vi "STP_23 - three_multiAO+dynamics+multifreq.vi"() -> ()   [LabVIEW 2020]
uses:
  <vilib>/Utility/error.llb/DialogType.ctl
  <vilib>/measure/NI_MABase.lvlib
  C:/Program Files/National Instruments/LabVIEW 2010/resource/objmgr/daqmx.rc
  <vilib>/Platform/TimedLoop/XDataNode/XDataNode.xnode
  <vilib>/Platform/TimedLoop/XDataNode/nitl_modes.ctl
  <vilib>/Platform/TimedLoop/XDataNode/XDNodeRunTimeDep.lvlib
  <vilib>/Platform/TimedLoop/XDataNode/wakeup.ctl
  <vilib>/Platform/TimedLoop/XDataNode/timing_clust.ctl
  <vilib>/measure/NI_MAPro.lvlib
  <vilib>/Math Plots/2D Math Plots/2D Compass/2D Compass Datatype/2D Compass Datatype.lvclass
  <vilib>/Math Plots/2D Math Plots/2D Compass/2D Compass Datatype/Public/Plot Helper (Vector).vi
  <vilib>/Analysis/NI_AALBase.lvlib
  <vilib>/Analysis/NI_AALPro.lvlib
  <vilib>/measure/matone.llb/Extract Single Tone Information 1 Chan.vi
  <vilib>/DAQmx/write.llb/DAQmx Write (Analog 1D Wfm NChan NSamp).vi
  <vilib>/DAQmx/configure/timing.llb/DAQmx Timing (Sample Clock).vi
  <vilib>/DAQmx/create/timing.llb/DAQmx Create Timing Source (Frequency).vi
  <vilib>/DAQmx/write.llb/DAQmx Write (Analog 2D DBL NChan NSamp).vi
  <vilib>/Instr/_visa.llb/VISA Configure Serial Port (Instr).vi
  <vilib>/DAQmx/create/channels.llb/DAQmx Create Channel (AO-Voltage-Basic).vi
  <vilib>/Math Plots/2D Math Plots/2D Compass/2D Compass XCtrl/2D Compass.xctl
panel:
  in  "Multi-freq. ?":bool
  in  "tones":T1(array[cluster])=[{"frequency"=100.0, "amplitude"=0.1, "phase"=210.0}, {"frequency"=200.0, "amplitude"=0.1, "phase"=39.0}, {"frequency"=250.0, "amplitude"=0.1, "phase"=30.0}, {"frequency"=300.0, "amplitude"=0.1, "phase"=60.0}, {"frequency"=350.0, "amplitude"=0.1, "phase"=184.0}, {"frequency"=400.0, "amplitude"=0.1, "phase"=35.0}] {"phase" format="%.2p"; "amplitude" format="%0.2p"; "frequency" format="%.4p"}
  out "rocof0":dbl[](array[numeric])
  out "rocof1":dbl[](array[numeric])
  out "ROCOF measured":dbl[](array[numeric])
  out "ROCOF reference":dbl[](array[numeric])
  out "Media":dbl
  in  "stop":bool
  out "Frequency reference":dbl[](array[numeric])
  out "Frequency measured":dbl[](array[numeric])
  out "Angle reference":dbl[](array[numeric])
  out "Angle measured":dbl[](array[numeric])
  out "Voltage reference":dbl[](array[numeric])
  out "Voltage measured":dbl[](array[numeric])
  out "freq1":dbl[](array[numeric])
  out "freq0":dbl[](array[numeric])
  out "magnitude1":dbl[](array[numeric])
  out "magnitude0":dbl[](array[numeric])
  in  "last amp":dbl
  out "phases0":dbl[](array[numeric])
  out "phases1":dbl[](array[numeric])
  out "initialized array":dbl[](array[numeric])
  out "Sine phase":dbl
  in  "Tab Control":T2(tab)
  out "Interf.\nAmplitude (%)":dbl
  out "Interf.\nFrequency (Hz)":dbl
  out "Amplitude (%)":dbl
  out "Harmonic order":i32
  out "reset\nphase?":bool
  out "Samples":dbl
  out "Frequency (Hz)":dbl
  out "Phase (deg)":dbl format="%.4f"
  out "Amplitude (V)":dbl format="%.4g"
  in  "Tab Control 3":T3(tab)
  in  "Interference":bool
  in  "Interf. Frequency":dbl caption="Frequency"
  in  "Interf. Amplitude":dbl caption="Amplitude (%)"
  in  "Amplitude (%)":dbl=10.0
  in  "Order":i32=2
  in  "Harmonics":bool
  in  "phase 2":dbl
  in  "duty cycle (%)":dbl=5.0
  in  "Pulse frequency":dbl=25.0
  in  "Noise":bool
  in  "Amplitude":dbl format="%.7f"
  in  "reset signal":bool
  in  "Phase":dbl format="%#.4f"
  in  "Frequency":dbl=50.0 format="%#.4f"
  in  "Offset":dbl=1.5 format="%#.4f"
  in  "Amplitude":dbl=1.25 format="%#.4f"
  in  "Steps":dbl=50.0
  in  "Save without\nvariation":bool
  in  "Amp. (%) 4":dbl=10.0 caption="Amplitude (%)"
  in  "Frequency\ninterval 2":dbl=0.25 caption="Frequency\ninterval"
  in  "Final freq. 2":dbl=51.25 caption="Final freq."
  in  "Initial freq. 2":dbl=48.75 caption="Initial freq."
  in  "Interference\nauto variation":bool
  in  "Amp. (%) 3":dbl=10.0 caption="Amplitude (%)"
  in  "Order\ninterval":i32=1
  in  "Final order":i32=50
  in  "Initial order":i32=2
  in  "Harmonics\nauto variation":bool
  in  "Frequency\ninterval":dbl=0.1 format="%.4f"
  in  "Final freq.":dbl=55.1 format="%.4f"
  in  "Initial freq.":dbl=45.0 format="%.4f"
  in  "Freq. auto\nvariation":bool
  in  "Phase\ninterval":dbl=10.0 format="%.4f"
  in  "Final phase":dbl=180.0 format="%.4f"
  in  "Initial phase":dbl=-180.0 format="%.4f"
  in  "Phase auto\nvariation":bool
  in  "Amplitude\ninterval":dbl=0.1 format="%.4f"
  in  "Initial ampl.":dbl=0.5 format="%.4f"
  in  "Final ampl.":dbl=6.0 format="%.4f"
  in  "Ampl. auto\nvariation":bool
  in  "Modulation tests?":bool
  in  "Final fmod":dbl=2.2
  in  "fmod interval":dbl=0.2
  in  "Initial fmod":dbl
  in  "Modulation\nauto variation":bool
  in  "Select test type":T4(ring)
  in  "Ramp test?":bool
  in  "ka":dbl=0.1
  in  "kx":dbl=0.1
  out "fmod (Hz)":dbl
  in  "fmod":dbl
  in  "Signal generation":bool=TRUE
  in  "File name":path=path "teste.txt"
  in  "Data save":bool
  in  "Boolean":bool
  in  "step time (s)":i32=2
  out "step?":bool
  out "Cycle visualization":dbl[](graph)
  in  "Boolean 3":bool
  out "Phasors visualization":refnum<class "2D Plot Datatype.lvclass">[](xcontrol) caption="2D Compass"
  in  "Directory":path=path "D:/Resultados"
  in  "Sampling rate":dbl=200000.0
  in  "frames per second":dbl=25.0
  in  "Porta":refnum<visa-resource-name>="COM5"
  in  "baud rate (kB)":u32=115200
  in  "data bits (8)":u16=8
  in  "timeout (ms)":u32=5000
  in  "parity (0:none)":enum16{"None", "Odd", "Even", "Mark", "Space"}(ring)
  in  "flow control (0:none)":u16(ring) items=["None", "XON/XOFF", "RTS/CTS", "XON/XOFF & RTS/CTS", "DTR/DSR", "XON/XOFF & DTR/DSR"]
  in  "stop bits (10: 1 bit)":u16(ring)=10 items=["1.0"=10, "1.5"=15, "2.0"=20]
  in  "Serial communication":bool=TRUE
  out "read buffer":string
  out "data":sgl[](array[numeric])
  in  "byte count":u32=16
  in  "Interference 2":bool caption="Interference"
  in  "amplitude":dbl=1.0 caption="Amp. (%)" format="%#.4p"
  in  "Interf. Frequency 2":dbl=10.0 caption="Frequency (Hz)"
  in  "Harmonics 2":bool caption="Harmonics"
  in  "Amp. (%) 2":dbl caption="Amp. (%)"
  in  "Order 2":i32=2 caption="Order"
  out "Frequency":dbl
  in  "Offset 2":dbl=1.5 caption="Offset"
  out "Phase (degrees) 2":dbl caption="Phase (°)" format="%.4f"
  in  "Amplitude 2":dbl=1.25 caption="Amplitude"
  in  "Frequency 2":dbl=50.0 caption="Frequency"
  in  "Phase 2":dbl caption="Phase"
  in  "reset signal 2":bool caption="reset\nsignal"
  in  "Frequency\noff-set":dbl
  in  "Magnitude\noff-set":dbl
  in  "Magnitude\ncoefficient":dbl=1.0
  in  "Angle\noff-set":dbl
  out "mean rocof":dbl caption="ROCOF (Hz/s)" format="%.8g"
  out "max rocof":dbl caption="ROCOF (Hz/s)" format="%.8g"
  out "mean freq":dbl caption="Frequency (Hz)" format="%.8g"
  out "mean tve":dbl caption="TVE (%)" format="%.8g"
  out "mean phase":dbl caption="Phase (º)" format="%.8g"
  out "mean dev":dbl caption="Magnitude (%)" format="%.8g"
  out "max magnitude":dbl caption="Magnitude (%)" format="%.8g"
  out "max tve":dbl caption="TVE (%)" format="%.8g"
  out "max freq":dbl caption="Frequency (Hz)" format="%.8g"
  out "max phase":dbl caption="Phase (º)" format="%.8g"
  in  "Tab Control 2":T5(tab)
  out "Magnitude measures (V)":dbl[][](graph)
  in  "?":bool
  in  "RMS?":bool=TRUE
  out "Phase measures (º)":dbl[][](graph)
  in  "?":bool
  in  "Fase ref":enum16{"R", "S", "T"}(ring)
  out "Frequency measures (Hz)":dbl[][](graph)
  in  "?":bool
  out "ROCOF (Hz/s)":dbl[][](graph)
  in  "?":bool
  in  "?":bool
  out "Phase measures (º) 2":dbl[](graph)
  in  "Index component":i32
  out "Iteration Duration 2":i64
  out "Finished Late? [i-1]":bool
  out "Iteration Duration":i64
  out "Iteration Duration 3":i64
  # "Synchrophasors Test Platform"
  # "A real-time platform for PMU development."
  # "(editar no diagrama de blocos, junto com os dados recebidos)"
  # "Actual generation"
  # "PPS parameters"
  # "Noise"
  # "Sinusoid parameters"
  # "IEEE 754 conversion"
  # "(tamanho do frame)"
  # "Max errors:"
  # "Mean errors:"
  # "Signal generation parameters:"
  # "On-line corrections (received data):"
  # "This is a project developed by Flavio Lori Grando, during Masters in Electrical Engineering Graduate Program (PPGEE) of Federal University of Technology - Paraná, Brazil.\n\nContact: flavio.grando.eng@gmail.com"
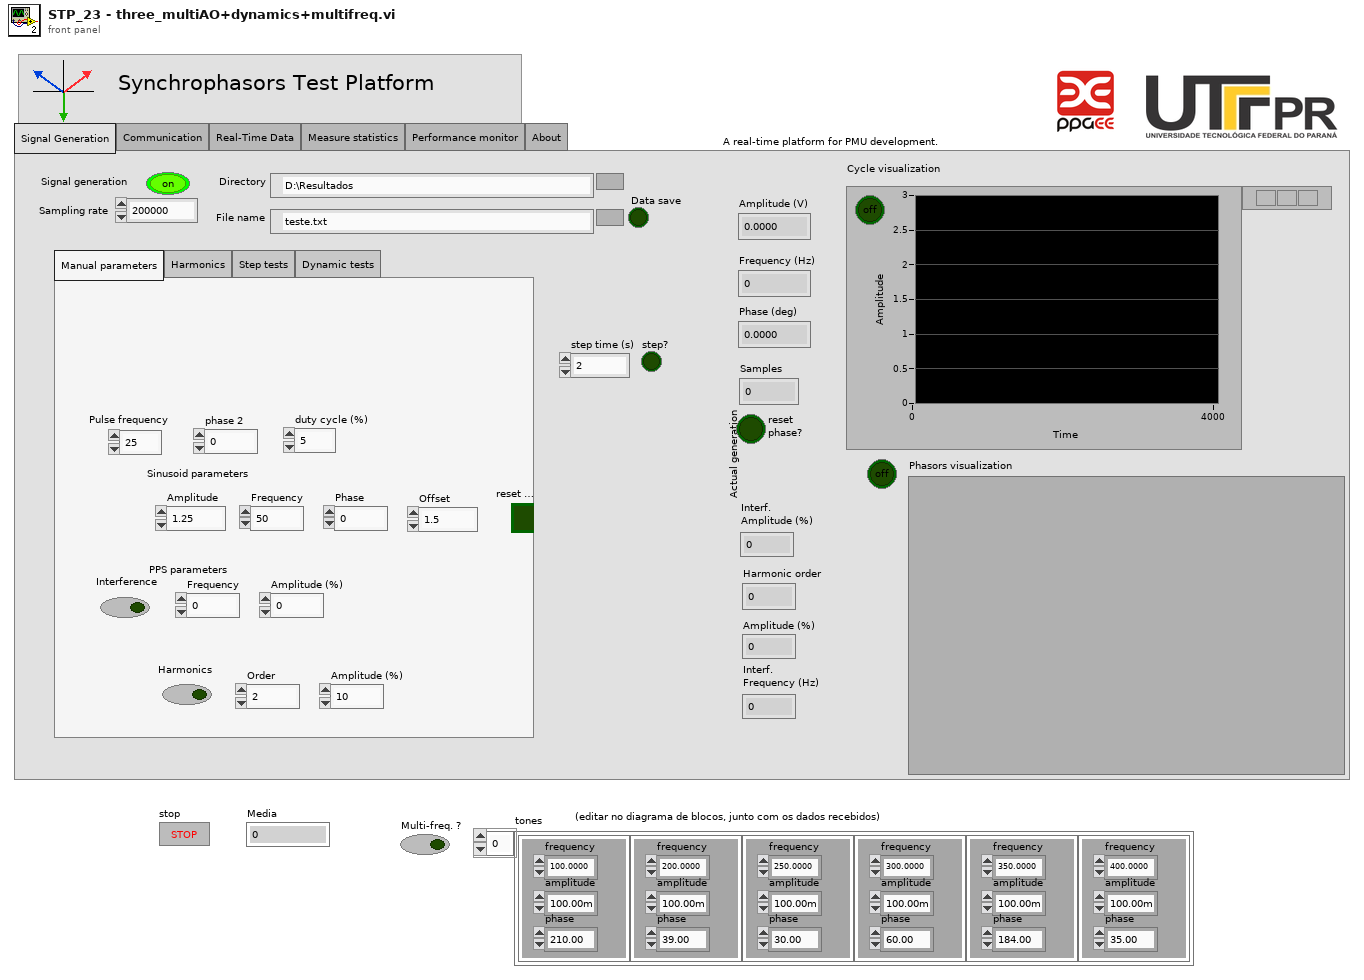
[diagram p1: front panel]
types:
  T1 = cluster{"frequency":dbl, "amplitude":dbl, "phase":dbl}[]
  T2 = enum32{"Signal Generation", "Communication", "Real-Time Data", "Measure statistics", "Performance monitor", "About"}
  T3 = enum32{"Manual parameters", "Harmonics", "Step tests", "Dynamic tests"}
  T4 = enum16{"Amplitude modulation", "Phase modulation", "Frequency ramp"}
  T5 = enum32{"Magnitude", "Phase", "Frequency", "ROCOF", "Phase deviation"}
  T6 = enum16{"Sine Wave", "Triangle Wave", "Square Wave", "Sawtooth Wave"}
  T7 = typedef "XDNodeRunTimeDep.lvlib/nitl_modes.ctl" = enum32{"No Change", "Process missed periods, maintain original phase", "Discard missed periods, maintain original phase", "Process missed periods, ignore original phase", "Discard missed periods, ignore original phase"}
  T8 = typedef "XDNodeRunTimeDep.lvlib/timing_clust.ctl" = cluster{"Expected End [f-1]":u64, "Actual End [f-1]":u64, "Finished Late? [f-1]":bool, "Expected End [i-1]":u64, "Actual End [i-1]":u64, "Finished Late? [i-1]":bool, "Expected Start [i]":u64, "Actual Start [i]":u64, "Expected Start [f]":u64, "Actual Start [f]":u64, "Source Name":string, "Structure Name":string, "Period":i64, "Deadline":i64, "Offset":i64, "Start":i64, "Priority":i32, "Timeout":i32, "Mode":T7, "Wakeup Reason":T9, "Error":errorcluster, "Source Type":string, "Secondary Source Type":string, "Global End Time":u64, "Global Start Time":u64, "Frame Duration":u64, "Iteration Duration":u64, "Assigned CPU":i32, "I/O Scan Engine Mode":u32}
  T9 = typedef "XDNodeRunTimeDep.lvlib/wakeup.ctl" = enum32{"Normal", "Aborted", "Asynchronous wakeup", "Timing source error", "Timed loop error", "Timeout"}
  T10 = typedef "DialogType.ctl" = u16
  T11 = cluster{"Sampling rate":dbl, "Sampling rate":dbl}
  T12 = cluster{"frequency":dbl, "amplitude":dbl, "phase":dbl}
  T13 = enum16{"open", "replace", "create", "open or create", "replace or create", "replace or create with confirmation"}
  T14 = cluster{"max ref":dbl, "min ref":dbl, "mean ref":dbl, "max dev":dbl, "min dev":dbl, "mean dev":dbl, "max meas":dbl, "min meas":dbl, "mean meas":dbl}
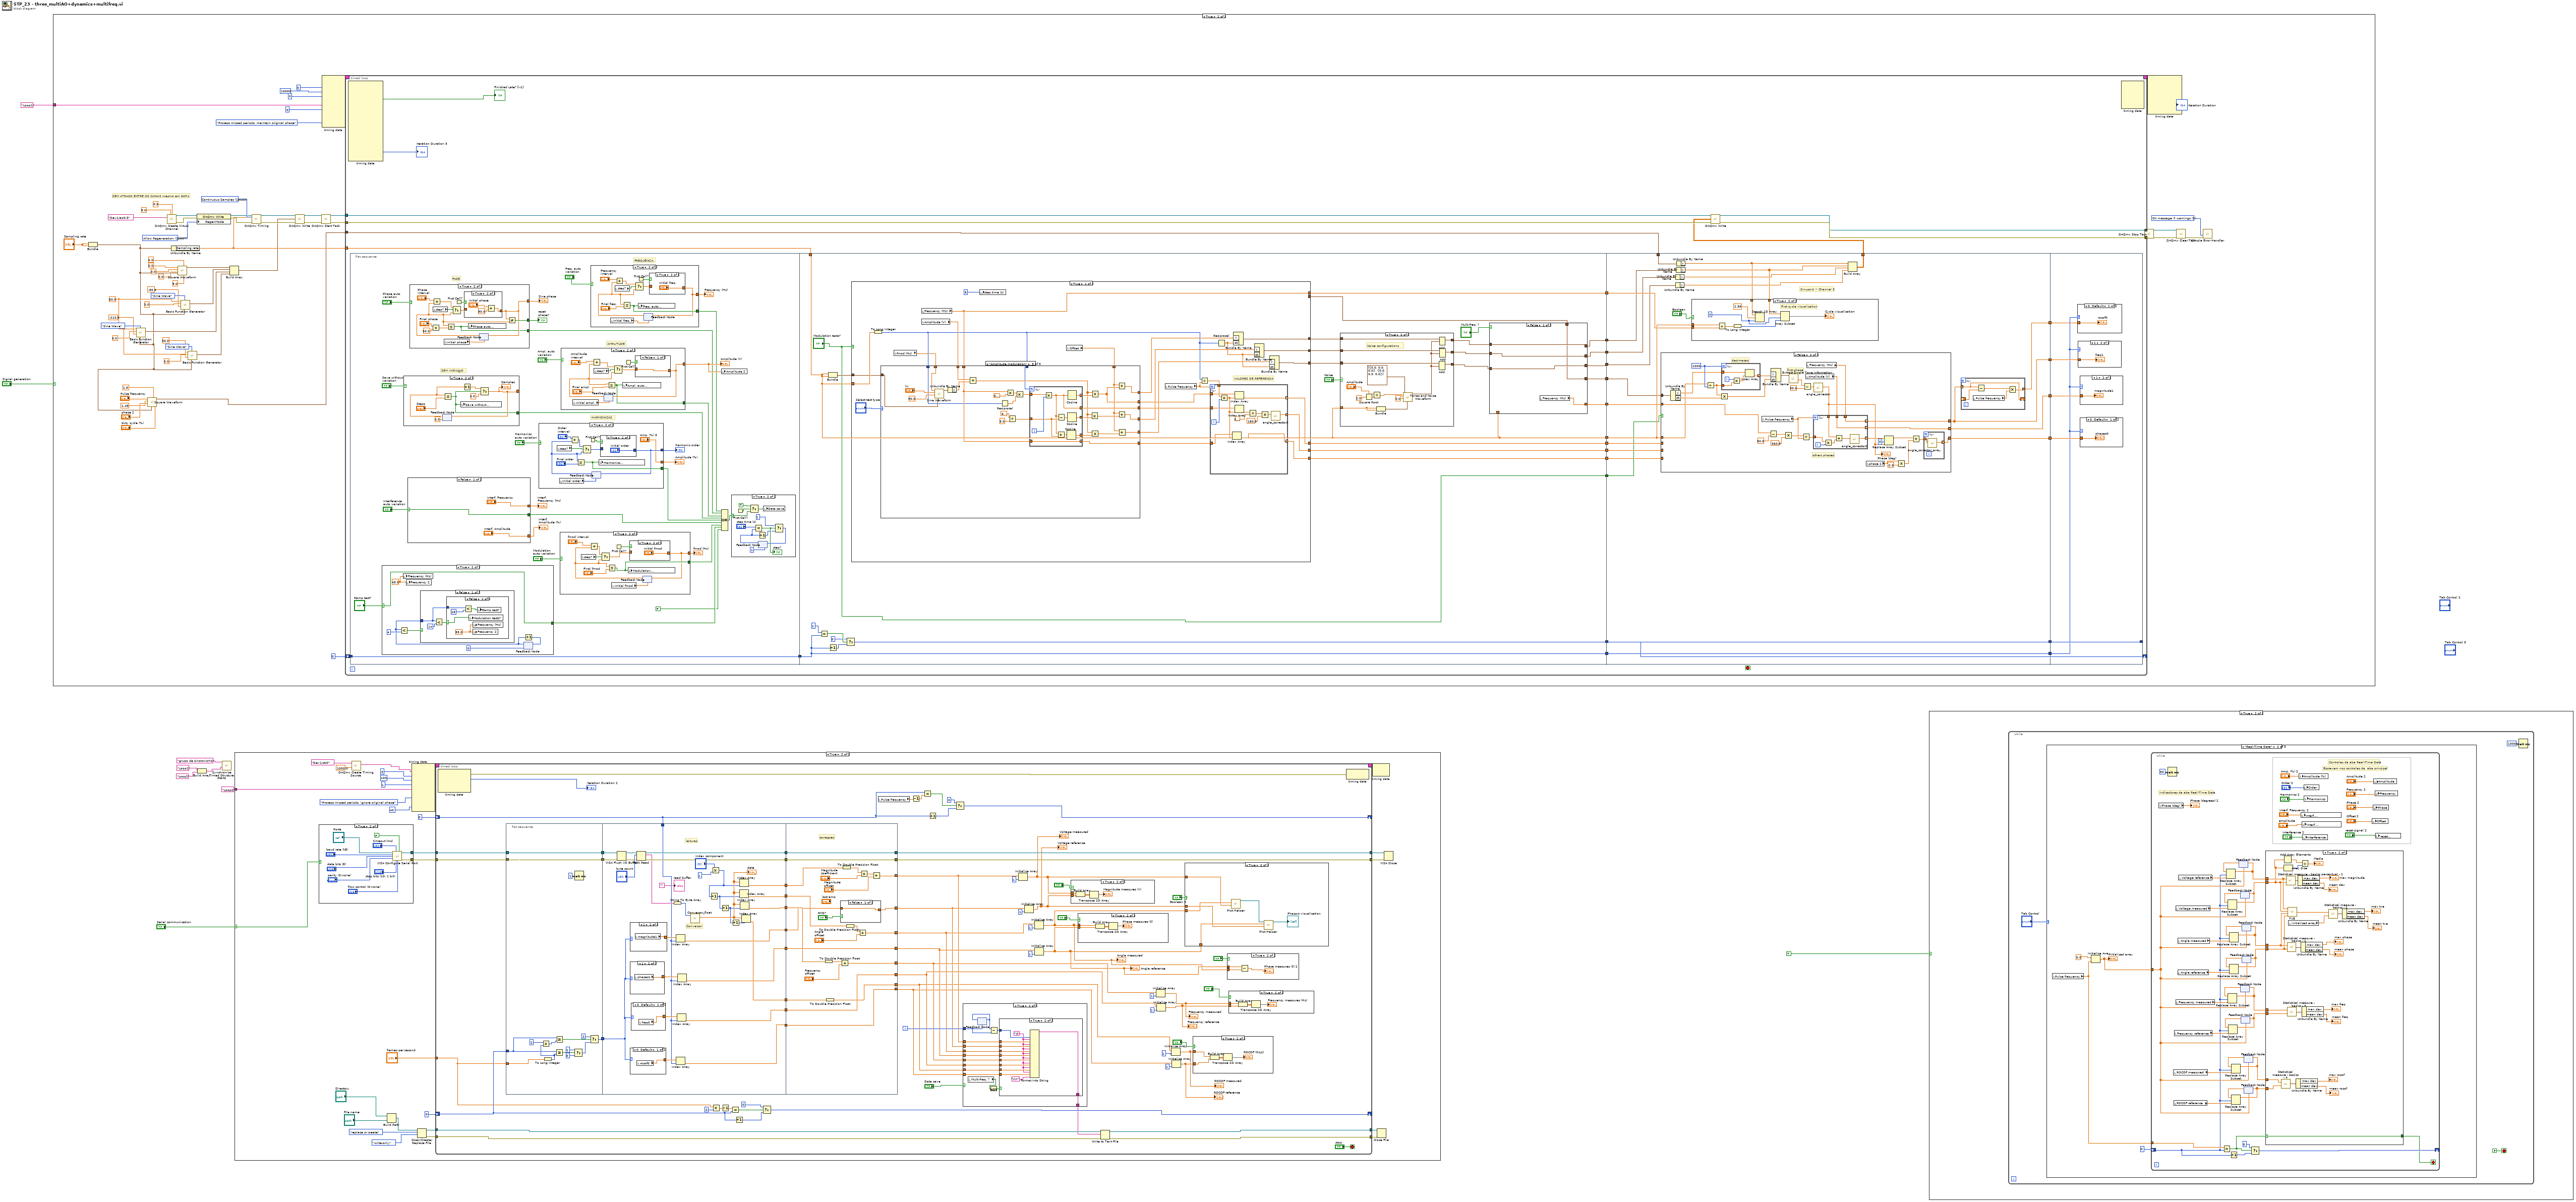
[diagram p0: block diagram]
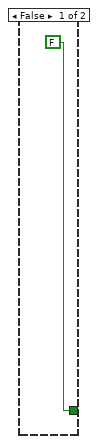
[diagram p4: hidden frame]
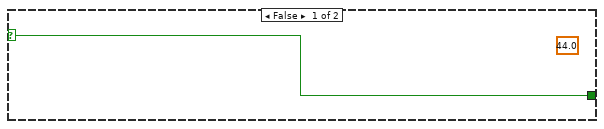
[diagram p7: hidden frame]
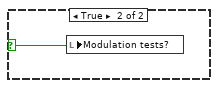
[diagram p8: hidden frame]
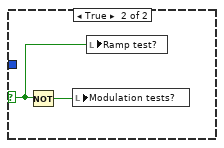
[diagram p9: hidden frame]
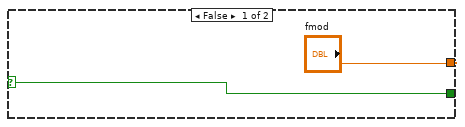
[diagram p10: hidden frame]
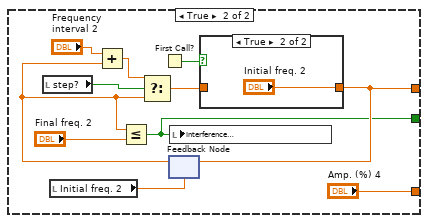
[diagram p12: hidden frame]
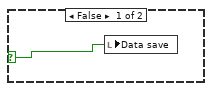
[diagram p14: hidden frame]
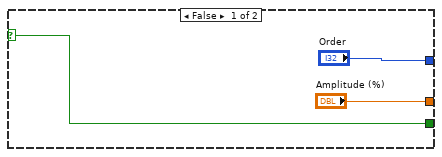
[diagram p15: hidden frame]
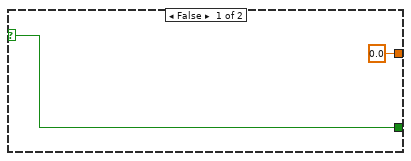
[diagram p17: hidden frame]
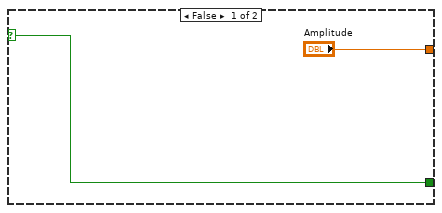
[diagram p18: hidden frame]
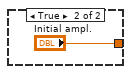
[diagram p19: hidden frame]
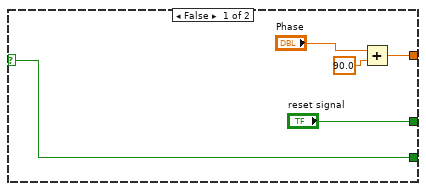
[diagram p20: hidden frame]
diagram:
  n1 = case shown="True" "Signal generation" {
    tunnel: "Loop1" -> [_ w33]
    frame False {
    }
    frame True {
      w20 = 60.0 ("frequency")
      w61 = 10097 items=["Allow Regeneration"=10097, "Do Not Allow Regeneration"=10158] ("RegenMode")
      w64 = 10123 items=["Finite Samples"=10178, "Continuous Samples"=10123] ("sample mode")
      w65 = T10 3 items=["no dialog", "OK message", "continue or stop message", "OK message + warnings", "continue/stop + warnings"] ("type of dialog (OK msg:1)")
      # "SEM ATRASO ENTRE OS CANAIS mesmo em 60Hz"
      n2 = Bundle("Sampling rate"="Sampling rate", "Sampling rate"="Sampling rate") -> (w11:T11)  [unwired: 1 in]
      n3 = call <vilib>:"Basic Function Generator.vi"("sampling info"=w11, "signal type"=T6."Sine Wave" ("signal type 4"), "phase"=-210.0 ("offset 4"), "amplitude"=0.0 ("amplitude 3"), "frequency"=w20) -> ("signal out"=w25:waveform(dbl))  [unwired: 4 in, 2 out]
      n4 = call <vilib>:"Square Waveform.vi"("duty cycle (%)"="duty cycle (%)", "offset"=1.5, "sampling info"=w11, "phase"="phase 2", "amplitude"=1.45, "frequency"="Pulse frequency") -> ("signal out"=w29:waveform(dbl))  [unwired: 4 in, 1 out]
      n5 = call-poly <vilib>:"DAQmx Create Virtual Channel.vi"("maximum value"=3.0 ("Maximum Value"), "minimum value"=0.0 ("Minimum Value"), "physical channels"=tag "Dev1/ao0:3" ("Physical Channel")) -> ("task out"=w40:refnum<k21>, "error out"=w41:errorcluster)  [unwired: 11 in]
      n6 = Unbundle By Name(w11) -> ("Sampling rate"=w10:dbl)
      n7 = call <vilib>:"Square Waveform.vi"("duty cycle (%)"=5.0, "offset"=0.0, "sampling info"=w11, "phase"=0.0, "amplitude"=0.0, "frequency"=0.0) -> ("signal out"=w31:waveform(dbl))  [unwired: 4 in, 1 out]
      n8 = call <vilib>:"Basic Function Generator.vi"("sampling info"=w11, "signal type"=T6."Sine Wave" ("signal type 4"), "phase"=-90.0 ("offset 4"), "amplitude"=0.0 ("amplitude 3"), "frequency"=w20) -> ("signal out"=w32:waveform(dbl))  [unwired: 4 in, 2 out]
      n9 = call <vilib>:"Basic Function Generator.vi"("sampling info"=w11, "signal type"=T6."Sine Wave" ("signal type 4"), "phase"=30.0 ("offset 4"), "amplitude"=0.0 ("amplitude 3"), "frequency"=w20) -> ("signal out"=w21:waveform(dbl))  [unwired: 4 in, 2 out]
      n10 = property class="DAQmx Write"(reference=w40, error in=w41, "RegenMode"=w61) -> (reference out=w14:refnum<k21>, error out=w62:errorcluster)
      n11 = Build Array(w31, w32, w25, w21) -> (w34:waveform(dbl)[])
      n12 = call-poly <vilib>:"DAQmx Timing.vi"("task/channels in"=w14, "sample mode"=w64, "rate"=w10, "error in"=w62) -> ("task out"=w36:refnum<k21>, "error out"=w35:errorcluster)  [unwired: 10 in]
      n13 = call-poly <vilib>:"DAQmx Write.vi"("task/channels in"=w36, "data"=w34, "error in"=w35) -> ("task out"=w45:refnum<k21>, "error out"=w46:errorcluster)  [unwired: 10 in, 1 out]
      n14 = call <vilib>:"DAQmx Start Task.vi"("task/channels in"=w45, "error in"=w46) -> ("task out"=w37:refnum<k21>, "error out"=w38:errorcluster)  [unwired: 12 in]
      n15 = node-c288(i64 0 ("Period"), 10000 ("Priority"), 0 ("Processor"), w33, i64 0 ("Deadline"), nitl_modes."Process missed periods, maintain original phase" ("Mode")) -> (w69:T8)  [unwired: 4 in]
      n16 = timed-loop {
        tunnel: w37 -> [w76]
        tunnel: [w92] -> w54
        tunnel: [w91] -> w53
        timing: w69 -> [_]
        timing-out: [_] -> w68
        shift-right: [w99] -> _
        shift-left: 0 -> [w80]
        tunnel: w38 -> [w93]
        tunnel: w29 -> [w75]
        tunnel: w10 -> [w72]
        stop <- _ stop-if-true
        n17 = node-c288() -> (→"Finished Late? [i-1]":bool, →"Iteration Duration 3":i64)  [unwired: 1 in, 15 out]
        n18 = flat-sequence {
          tunnel: w80 -> [w123]
          tunnel: [w123] -> w89
          tunnel: [w285] -> w90
          tunnel: w89 -> [w284]
          tunnel: [w284] -> w88
          tunnel: [w268] -> w87
          tunnel: [w290] -> w86
          tunnel: [w274] -> w84
          tunnel: [w273] -> w83
          tunnel: [w275] -> w82
          tunnel: [w279] -> w79
          tunnel: [w277] -> w78
          tunnel: [w278] -> w77
          tunnel: ["Modulation tests?"] -> w73
          tunnel: w72 -> [w268]
          tunnel: [w267] -> w71
          tunnel: [w266] -> w70
          tunnel: [w614] -> w98
          tunnel: [w612] -> w97
          tunnel: [w606] -> w96
          tunnel: [w594] -> w95
          tunnel: w90 -> [w614]
          tunnel: w88 -> [w613]
          tunnel: [w613] -> w94
          tunnel: [w609] -> w74
          tunnel: w87 -> [w611]
          tunnel: w86 -> [w610]
          tunnel: [w593] -> w85
          tunnel: w84 -> [w605]
          tunnel: w83 -> [w604]
          tunnel: w82 -> [w599]
          tunnel: w79 -> [w608]
          tunnel: w78 -> [w595]
          tunnel: w77 -> [w607]
          tunnel: w75 -> [w598]
          tunnel: w73 -> [w596]
          tunnel: w71 -> [w592]
          tunnel: w70 -> [w591]
          tunnel: w98 -> [w684]
          tunnel: [w684] -> w99
          tunnel: w97 -> [w683]
          tunnel: w96 -> [w682]
          tunnel: w95 -> [w681]
          tunnel: w94 -> [w680]
          tunnel: w85 -> [w679]
          frame #0 {
            # "HARMONICAS"
            # "SEM VARIA敲O"
            # "FASE"
            # "FREQUÊNCIA"
            # "AMPLITUDE"
            n19 = case shown="True" "Ramp test?" {
              selector: "Ramp test?" -> [w129 w131]
              tunnel: [w129 w131] -> w102
              frame False {
                (unwired) 44.0 ("Initial freq. 3")
              }
              frame True {
                w130 = 45.0 ("Frequency")
                n20 = local write "Frequency (Hz)"(w130) -> ()
                n21 = local write "Frequency 2"(w130) -> ()
                n22 = feedback #1(0) -> (w133:i32)
                n23 = Less?(x=w133, y=4) -> (x < y?=w132:bool)
                n24 = case shown="False" w132 {
                  selector: w132 -> [_ w146]
                  tunnel: w133 -> [w138 _]
                  frame False {
                    n25 = Less?(x=w138, y=14) -> (x < y?=w137:bool)
                    n26 = case shown="False" w137 {
                      selector: w137 -> [w140 w145]
                      tunnel: w138 -> [w143 _]
                      frame False {
                        w141 = 55.0 ("Frequency")
                        n27 = Less?(x=w143, y=18) -> (x < y?=w142:bool)
                        n28 = local write "Modulation tests?"(w140) -> ()
                        n29 = local write "Frequency (Hz)"(w141) -> ()
                        n30 = local write "Frequency 2"(w141) -> ()
                        n31 = local write "Ramp test?"(w142) -> ()
                      }
                      frame True {
                        n32 = local write "Modulation tests?"(w145) -> ()
                      }
                    }
                  }
                  frame True {
                    n33 = Not(x=w146) -> (.not. x?=w147:bool)
                    n34 = local write "Modulation tests?"(w147) -> ()
                    n35 = local write "Ramp test?"(w146) -> ()
                  }
                }
                n36 = Increment(x=w133) -> (x+1=w135:i32)
                n37 = feedback-in #1(w135) -> ()
              }
            }
            n38 = case shown="True" "Save without\nvariation" {
              selector: "Save without\nvariation" -> [w206 _]
              tunnel: [0.0 ("f") w209] -> _
              tunnel: [w206 w208] -> w117
              frame False {
              }
              frame True {
                n39 = feedback #2(0.0 ("f")) -> (w211:dbl)
                n40 = Less Or Equal?(x=w211, y="Steps") -> (x <= y?=w208:bool)
                n41 = local write "Save without\nvariation"(w208) -> ()
                n42 = Increment(x=w211) -> (x+1=w213:dbl)
                n43 = Select(t=w213, s=w208, f=0.0) -> (s? t:f=w209:dbl)
                "Samples" <- w209
                n44 = feedback-in #2(w209) -> ()
              }
            }
            n45 = case shown="False" "Interference\nauto variation" {
              selector: "Interference\nauto variation" -> [w162 _]
              tunnel: ["Interf. Frequency" w171] -> w109
              tunnel: ["Interf. Amplitude" "Amp. (%) 4"] -> w108
              tunnel: [w162 w165] -> w107
              frame False {
              }
              frame True {
                n46 = local read "step?"() -> (w168:bool)
                n47 = local read "Initial freq. 2"() -> (w172:dbl)
                n48 = First Call?() -> (First Call?: T/F=w175:bool)
                n49 = feedback #3(w172) -> (w167:dbl)
                n50 = Add(x="Frequency\ninterval 2", y=w167) -> (x+y=w169:dbl)
                n51 = Less Or Equal?(x=w167, y="Final freq. 2") -> (x <= y?=w165:bool)
                n52 = Select(t=w169, s=w168, f=w167) -> (s? t:f=w174:dbl)
                n53 = local write "Interference\nauto variation"(w165) -> ()
                n54 = case shown="True" w175 {
                  tunnel: [w176 "Initial freq. 2"] -> w171
                  tunnel: w174 -> [w176 _]
                  frame False {
                  }
                  frame True {
                  }
                }
                n55 = feedback-in #3(w171) -> ()
              }
            }
            "Interf.\nFrequency (Hz)" <- w109
            "Interf.\nAmplitude (%)" <- w108
            n56 = case shown="True" "Phase auto\nvariation" {
              selector: "Phase auto\nvariation" -> [w229 _]
              tunnel: ["reset signal" w244] -> w128
              tunnel: [w231 w243] -> w118
              tunnel: [w229 w238] -> w115
              frame False {
                n57 = Add(x="Phase", y=90.0) -> (x+y=w231:dbl)
              }
              frame True {
                n58 = Add(x="Final phase", y=90.0) -> (x+y=w240:dbl)
                n59 = local read "step?"() -> (w234:bool)
                n60 = local read "Initial phase"() -> (w242:dbl)
                n61 = First Call?() -> (First Call?: T/F=w245:bool)
                n62 = feedback #4(w242) -> (w236:dbl)
                n63 = Add(x="Phase\ninterval", y=w236) -> (x+y=w235:dbl)
                n64 = Less Or Equal?(x=w236, y=w240) -> (x <= y?=w238:bool)
                n65 = Select(t=w235, s=w234, f=w236) -> (s? t:f=w237:dbl)
                n66 = case shown="True" w245 {
                  tunnel: [w247 w248] -> w243
                  tunnel: w237 -> [w247 _]
                  frame False {
                  }
                  frame True {
                    n67 = Add(x="Initial phase", y=90.0) -> (x+y=w248:dbl)
                  }
                }
                n68 = local write "Phase auto\nvariation"(w238) -> ()
                n69 = feedback-in #4(w243) -> ()
                n70 = Not Equal?(x=w243, y=w236) -> (x != y?=w244:bool)
              }
            }
            "Sine phase" <- w118
            "reset\nphase?" <- w128
            n71 = case shown="True" "Harmonics\nauto variation" {
              selector: "Harmonics\nauto variation" -> [w191 _]
              tunnel: ["Order" w197] -> w113
              tunnel: [w191 w198] -> w111
              tunnel: ["Amplitude (%)" "Amp. (%) 3"] -> w112
              frame False {
              }
              frame True {
                n72 = local read "step?"() -> (w200:bool)
                n73 = local read "Initial order"() -> (w202:i32)
                n74 = First Call?() -> (First Call?: T/F=w199:bool)
                n75 = feedback #5(w202) -> (w195:i32)
                n76 = Add(x="Order\ninterval", y=w195) -> (x+y=w194:i32)
                n77 = Less Or Equal?(x=w195, y="Final order") -> (x <= y?=w198:bool)
                n78 = Select(t=w194, s=w200, f=w195) -> (s? t:f=w203:i32)
                n79 = local write "Harmonics\nauto variation"(w198) -> ()
                n80 = case shown="True" w199 {
                  tunnel: [w204 "Initial order"] -> w197
                  tunnel: w203 -> [w204 _]
                  frame False {
                  }
                  frame True {
                  }
                }
                n81 = feedback-in #5(w197) -> ()
              }
            }
            "Harmonic order" <- w113
            "Amplitude (%)" <- w112
            n82 = case shown="True" "Modulation\nauto variation" {
              selector: "Modulation\nauto variation" -> [w149 _]
              tunnel: [w149 w152] -> w105
              tunnel: ["fmod" w151] -> w104
              frame False {
              }
              frame True {
                n83 = local read "step?"() -> (w158:bool)
                n84 = local read "Initial fmod"() -> (w150:dbl)
                n85 = First Call?() -> (First Call?: T/F=w159:bool)
                n86 = feedback #6(w150) -> (w155:dbl)
                n87 = Add(x="fmod interval", y=w155) -> (x+y=w157:dbl)
                n88 = Select(t=w157, s=w158, f=w155) -> (s? t:f=w153:dbl)
                n89 = Less Or Equal?(x=w155, y="Final fmod") -> (x <= y?=w152:bool)
                n90 = local write "Modulation\nauto variation"(w152) -> ()
                n91 = case shown="True" w159 {
                  tunnel: [w160 "Initial fmod"] -> w151
                  tunnel: w153 -> [w160 _]
                  frame False {
                  }
                  frame True {
                  }
                }
                n92 = feedback-in #6(w151) -> ()
              }
            }
            "fmod (Hz)" <- w104
            n93 = case shown="True" "Ampl. auto\nvariation" {
              selector: "Ampl. auto\nvariation" -> [w215 _]
              tunnel: ["Amplitude" w224] -> w122
              tunnel: [w215 w219] -> w116
              frame False {
              }
              frame True {
                n94 = local read "Initial ampl."() -> (w223:dbl)
                n95 = local read "step?"() -> (w220:bool)
                n96 = feedback #7(w223) -> (w218:dbl)
                n97 = Add(x="Amplitude\ninterval", y=w218) -> (x+y=w222:dbl)
                n98 = Less Or Equal?(x=w218, y="Final ampl.") -> (x <= y?=w219:bool)
                n99 = Select(t=w222, s=w220, f=w218) -> (s? t:f=w221:dbl)
                n100 = local write "Ampl. auto\nvariation"(w219) -> ()
                n101 = First Call?() -> (First Call?: T/F=w225:bool)
                n102 = case shown="False" w225 {
                  tunnel: [w227 "Initial ampl."] -> w224
                  tunnel: w221 -> [w227 _]
                  frame False {
                  }
                  frame True {
                  }
                }
                n103 = feedback-in #7(w224) -> ()
              }
            }
            "Amplitude (V)" <- w122
            n104 = case shown="True" "Freq. auto\nvariation" {
              selector: "Freq. auto\nvariation" -> [w252 _]
              tunnel: ["Frequency" w259] -> w120
              tunnel: [w252 w257] -> w114
              frame False {
              }
              frame True {
                n105 = local read "Initial freq."() -> (w258:dbl)
                n106 = local read "step?"() -> (w253:bool)
                n107 = First Call?() -> (First Call?: T/F=w261:bool)
                n108 = feedback #8(w258) -> (w254:dbl)
                n109 = Add(x="Frequency\ninterval", y=w254) -> (x+y=w255:dbl)
                n110 = Less Or Equal?(x=w254, y="Final freq.") -> (x <= y?=w257:bool)
                n111 = Select(t=w255, s=w253, f=w254) -> (s? t:f=w256:dbl)
                n112 = local write "Freq. auto\nvariation"(w257) -> ()
                n113 = case shown="True" w261 {
                  tunnel: [w263 "Initial freq."] -> w259
                  tunnel: w256 -> [w263 _]
                  frame False {
                  }
                  frame True {
                  }
                }
                n114 = feedback-in #8(w259) -> ()
              }
            }
            "Frequency (Hz)" <- w120
            n115 = local write "Amplitude 2"(w122) -> ()
            n116 = Compound Arithmetic op=OR(w114, w115, w116, w117, w111, w107, w105, w102, FALSE ("Boolean 2")) -> (w119:bool)
            n117 = case shown="True" w119 {
              selector: w119 -> [w178 w187]
              frame False {
                n118 = local write "Data save"(w178) -> ()
              }
              frame True {
                n119 = First Call?() -> (First Call?: T/F=w189:bool)
                n120 = Select(t=TRUE, s=w189, f=w187) -> (s? t:f=w186:bool)
                n121 = feedback #9(1 ("f")) -> (w179:i32)
                n122 = Equal?(x="step time (s)", y=w179) -> (x = y?=w182:bool)
                "step?" <- w182
                n123 = Increment(x=w179) -> (x+1=w180:i32)
                n124 = local write "Data save"(w186) -> ()
                n125 = Select(t=1 ("f"), s=w182, f=w180) -> (s? t:f=w185:i32)
                n126 = feedback-in #9(w185) -> ()
              }
            }
          }
          frame #1 {
            n127 = Equal?(x=1, y=w284) -> (x = y?=w289:bool)
            n128 = Bundle("Sampling rate"=w268, "Sampling rate"=w268) -> (w291:T11)  [unwired: 1 in]
            n129 = Increment(x=w284) -> (x+1=w287:i32)
            n130 = Select(t=0, s=w289, f=w287) -> (s? t:f=w285:i32)
            n131 = case shown="True" "Modulation tests?" {
              tunnel: w291 -> [w342 w521]
              tunnel: [w346 w537] -> w290
              tunnel: [w351 w519] -> w283
              tunnel: [w350 w520] -> w282
              tunnel: [w356 w518] -> w280
              tunnel: [_ w523] -> w265
              tunnel: w268 -> [w354 _]
              tunnel: [w345 _] -> w279
              tunnel: [w344 _] -> w278
              tunnel: [w335 _] -> w277
              frame True {
                # "VALORES DE REFERENCIA"
                n132 = To Long Integer(number=w354) -> (32bit integer=w348:i32)
                n133 = local read "fmod (Hz)"() -> (w343:dbl)
                n134 = local read "Frequency (Hz)"() -> (w346:dbl)
                n135 = local read "Amplitude (V)"() -> (w355:dbl)
                n136 = local write "step time (s)"(5) -> ()
                n137 = local read "Offset"() -> (w334:dbl)
                n138 = case shown="\"Amplitude modulation\"" "Select test type" {
                  tunnel: w355 -> [w368 w413 w493]
                  tunnel: w346 -> [w365 w411 w481]
                  tunnel: w348 -> [_ w416 w474]
                  tunnel: [w382 w402 w488] -> w336
                  tunnel: [w362 w408 w465] -> w339
                  tunnel: [w360 w403 w467] -> w341
                  tunnel: [w359 w405 w469] -> w340
                  tunnel: w348 -> [w364 _ w471]
                  tunnel: [w376 w415 w480] -> w337
                  tunnel: w343 -> [w374 _ w475]
                  tunnel: w342 -> [w375 _ w473]
                  tunnel: [w367 w419 w464] -> w338
                  tunnel: w334 -> [w358 w407 w468]
                  frame "Phase modulation" {
                    # "referencia"
                    n139 = call <vilib>:"Sine Waveform.vi"("sampling info"=w375, "phase"=-90.0, "amplitude"="ka", "frequency"=w374) -> ("signal out"=w378:waveform(dbl))  [unwired: 6 in, 1 out]
                    n140 = call <vilib>:"Sine Waveform.vi"("sampling info"=w375, "phase"=-180.0, "amplitude"="ka", "frequency"=w374) -> ("signal out"=w372:waveform(dbl))  [unwired: 6 in, 1 out]
                    n141 = Unbundle By Name(w378) -> ("Y"=w369:dbl[])
                    n142 = Unbundle By Name(w372) -> ("Y"=w371:dbl[])
                    n143 = Reciprocal(x=w364) -> (1/x=w366:dbl)
                    n144 = Multiply(x=w365, y=6.283185307179586) -> (x*y=w380:dbl)
                    n145 = Divide(x=6.283185307179586, y=3.0) -> (x/y=w385:dbl)
                    n146 = Multiply(x=w380, y=w366) -> (x*y=w381:dbl)
                    n147 = for {
                      N: w364 -> [_]
                      tunnel: w381 -> [w393]
                      tunnel: [w401] -> w388 mode=indexing
                      tunnel: [w390] -> w382 mode=indexing
                      tunnel: w385 -> [w398]
                      tunnel: [w397] -> w384 mode=indexing
                      tunnel: [w396] -> w383 mode=indexing
                      tunnel: w369 -> [w390] mode=indexing
                      tunnel: [w391] -> w367 mode=indexing
                      tunnel: w368 -> [w391]
                      i -> [w392]
                      n148 = Multiply(x=w393, y=w392) -> (x*y=w395:dbl)
                      n149 = Add(x=w395, y=w390) -> (x+y=w394:dbl)
                      n150 = Add(x=w394, y=w398) -> (x+y=w399:dbl)
                      n151 = Subtract(x=w394, y=w398) -> (x-y=w400:dbl)
                      n152 = Cosine(x=w399) -> (cos(x)=w397:dbl)
                      n153 = Cosine(x=w400) -> (cos(x)=w396:dbl)
                      n154 = Cosine(x=w394) -> (cos(x)=w401:dbl)
                    }
                    n155 = Multiply(x=w371, y=w374) -> (x*y=w377:dbl[])
                    n156 = Multiply(x=w368, y=w383) -> (x*y=w361:dbl[])
                    n157 = Multiply(x=w368, y=w384) -> (x*y=w357:dbl[])
                    n158 = Multiply(x=w368, y=w388) -> (x*y=w363:dbl[])
                    n159 = Subtract(x=w365, y=w377) -> (x-y=w376:dbl[])
                    n160 = Add(x=w358, y=w363) -> (x+y=w362:dbl[])
                    n161 = Add(x=w358, y=w357) -> (x+y=w359:dbl[])
                    n162 = Add(x=w358, y=w361) -> (x+y=w360:dbl[])
                  }
                  frame "Frequency ramp" {
                    w422 = u16 0 items=["2nd Order Central", "4th Order Central", "Forward", "Backward"] ("method")
                    w417 = 1 items=["none", "linear"] ("interpolation")
                    w428 = cluster{"Fs":dbl, "#s":dbl} {"Fs"=25000.0, "#s"=25000.0} ("sampling info")
                    n163 = case shown="True" TRUE {
                      tunnel: w416 -> [w438 w456]
                      tunnel: [w435 w453] -> w415
                      tunnel: w411 -> [w439 w451]
                      frame False {
                        n164 = First Call?() -> (First Call?: T/F=w441:bool)
                        n165 = feedback #10(w439) -> (w442:dbl)
                        n166 = Decrement(x=w442) -> (x-1=w440:dbl)
                        n167 = Select(t=w439, s=w441, f=w440) -> (s? t:f=w443:dbl)
                        n168 = feedback-in #10(w443) -> ()
                        n169 = Reciprocal(x=w438) -> (1/x=w436:dbl)
                        n170 = for {
                          N: w438 -> [_]
                          tunnel: w436 -> [w447]
                          tunnel: [w446] -> w444 mode=indexing
                          i -> [w445]
                          n171 = Multiply(x=w447, y=w445) -> (x*y=w446:dbl)
                        }
                        n172 = Subtract(x=w443, y=w444) -> (x-y=w437:dbl[])
                        n173 = Subtract(x=w437, y=w436) -> (x-y=w435:dbl[])
                      }
                      frame True {
                        w448 = 1.0 ("x")
                        n174 = First Call?() -> (First Call?: T/F=w458:bool)
                        n175 = feedback #11(w451) -> (w450:dbl)
                        n176 = Add(x=w448, y=w450) -> (x+y=w449:dbl)
                        n177 = Select(t=w451, s=w458, f=w449) -> (s? t:f=w457:dbl)
                        n178 = feedback-in #11(w457) -> ()
                        n179 = Reciprocal(x=w456) -> (1/x=w452:dbl)
                        n180 = for {
                          N: w456 -> [_]
                          tunnel: w452 -> [w463]
                          tunnel: [w460] -> w455 mode=indexing
                          tunnel: w448 -> [w459]
                          i -> [w462]
                          n181 = Multiply(x=w463, y=w462) -> (x*y=w461:dbl)
                          n182 = Multiply(x=w459, y=w461) -> (x*y=w460:dbl)
                        }
                        n183 = Add(x=w457, y=w455) -> (x+y=w454:dbl[])
                        n184 = Add(x=w452, y=w454) -> (x+y=w453:dbl[])
                      }
                    }
                    n185 = call <vilib>:"Formula Waveform.vi"("sampling info"=w428, "formula"="a*cos(w*t+pi(1)*t*t)", "amplitude"=w413, "frequency"=w411) -> ("signal out"=w433:waveform(dbl))  [unwired: 6 in, 1 out]
                    n186 = call <vilib>:"Formula Waveform.vi"("sampling info"=w428, "formula"="a*cos(w*t+pi(1)*t*t-pi(1)*2/3)", "amplitude"=w413, "frequency"=w411) -> ("signal out"=w430:waveform(dbl))  [unwired: 6 in, 1 out]
                    n187 = call <vilib>:"Formula Waveform.vi"("sampling info"=w428, "formula"="a*cos(w*t+pi(1)*t*t+2*pi(1)/3)", "amplitude"=w413, "frequency"=w411) -> ("signal out"=w429:waveform(dbl))  [unwired: 6 in, 1 out]
                    n188 = Unbundle By Name(w430) -> ("Y"=w425:dbl[])
                    n189 = Unbundle By Name(w429) -> ("Y"=w424:dbl[])
                    n190 = Unbundle By Name(w433) -> ("Y"=w426:dbl[])
                    n191 = Divide(x=1.0, y=w416) -> (x/y=w423:dbl)
                    n192 = call <vilib>:"Arbitrary Wave.vi"("interpolation"=w417, "Wave Table"=w426, "frequency"=w423, "samples"=w416) -> ("arbitrary wave"=w409:dbl[])  [unwired: 3 in, 2 out]
                    n193 = call <vilib>:"Arbitrary Wave.vi"("interpolation"=w417, "Wave Table"=w424, "frequency"=w423, "samples"=w416) -> ("arbitrary wave"=w406:dbl[])  [unwired: 3 in, 2 out]
                    n194 = call <vilib>:"Arbitrary Wave.vi"("interpolation"=w417, "Wave Table"=w425, "frequency"=w423, "samples"=w416) -> ("arbitrary wave"=w404:dbl[])  [unwired: 3 in, 2 out]
                    n195 = Divide(x=w409, y=w413) -> (x/y=w412:dbl[])
                    n196 = Inverse Cosine(1:w412) -> (0:w414:dbl[])
                    n197 = Initialize Array(w413, w416) -> (w419:dbl[])
                    n198 = call <vilib>:"Derivative x(t).vi"("method"=w422, "dt"=1e-05, "X"=w414) -> ("dX/dt"=w420:dbl[])  [unwired: 7 in, 1 out]
                    n199 = Sign(1:w420) -> (0:w418:dbl[])
                    n200 = Multiply(x=w414, y=w418) -> (x*y=w402:dbl[])
                    n201 = Add(x=w407, y=w409) -> (x+y=w408:dbl[])
                    n202 = Add(x=w407, y=w404) -> (x+y=w403:dbl[])
                    n203 = Add(x=w407, y=w406) -> (x+y=w405:dbl[])
                  }
                  frame "Amplitude modulation" {
                    n204 = call <vilib>:"Sine Waveform.vi"("sampling info"=w473, "phase"=90.0 ("phase in"), "amplitude"="kx", "frequency"=w475) -> ("signal out"=w477:waveform(dbl))  [unwired: 6 in, 1 out]
                    n205 = Unbundle By Name(w477) -> ("Y"=w476:dbl[])
                    n206 = Add(x=w493, y=w476) -> (x+y=w482:dbl[])
                    n207 = Reciprocal(x=w471) -> (1/x=w472:dbl)
                    n208 = Multiply(x=w481, y=6.283185307179586) -> (x*y=w491:dbl)
                    n209 = Divide(x=6.283185307179586, y=3.0) -> (x/y=w485:dbl)
                    n210 = Multiply(x=w491, y=w472) -> (x*y=w490:dbl)
                    n211 = for {
                      N: w474 -> [_]
                      tunnel: w490 -> [w501]
                      tunnel: [w502] -> w489 mode=indexing
                      tunnel: [w498] -> w488 mode=indexing
                      tunnel: w485 -> [w497]
                      tunnel: [w496] -> w484 mode=indexing
                      tunnel: [w495] -> w483 mode=indexing
                      tunnel: [w494] -> w480 mode=indexing
                      tunnel: w481 -> [w494]
                      i -> [w503]
                      n212 = Multiply(x=w501, y=w503) -> (x*y=w498:dbl)
                      n213 = Add(x=w498, y=w497) -> (x+y=w499:dbl)
                      n214 = Subtract(x=w498, y=w497) -> (x-y=w500:dbl)
                      n215 = Cosine(x=w499) -> (cos(x)=w496:dbl)
                      n216 = Cosine(x=w500) -> (cos(x)=w495:dbl)
                      n217 = Cosine(x=w498) -> (cos(x)=w502:dbl)
                    }
                    n218 = Multiply(x=w482, y=w483) -> (x*y=w466:dbl[])
                    n219 = Multiply(x=w482, y=w484) -> (x*y=w470:dbl[])
                    n220 = Multiply(x=w482, y=w489) -> (x*y=w464:dbl[])
                    n221 = Add(x=w468, y=w464) -> (x+y=w465:dbl[])
                    n222 = Add(x=w468, y=w466) -> (x+y=w467:dbl[])
                    n223 = Add(x=w468, y=w470) -> (x+y=w469:dbl[])
                  }
                }
                n224 = local read "Pulse frequency"() -> (w353:dbl)
                n225 = Divide(x=w348, y=w353) -> (x/y=w352:dbl)
                n226 = for {
                  N: w353 -> [_]
                  tunnel: w336 -> [w517]
                  tunnel: w352 -> [w515]
                  tunnel: [w508] -> w345 mode=indexing
                  tunnel: w338 -> [w509]
                  tunnel: [w507] -> w344 mode=indexing
                  tunnel: w337 -> [w506]
                  tunnel: [w504] -> w335 mode=indexing
                  i -> [w516]
                  n227 = Multiply(x=w515, y=w516) -> (x*y=w505:dbl)
                  n228 = Index Array(array=w506, index=w505) -> (element=w504:dbl)
                  n229 = Index Array(array=w517, index=w505) -> (element=w512:dbl)
                  n230 = Index Array(array=w509, index=w505) -> (element=w508:dbl)
                  n231 = Divide(x=w512, y=3.141592653589793) -> (x/y=w511:dbl)
                  n232 = Multiply(x=w511, y=180.0) -> (x*y=w510:dbl)
                  n233 = call "angle_corrector2.vi"("angle"=w510) -> ("angle corrected"=w507:dbl)  [unwired: 10 in]
                }
                n234 = Reciprocal(x=w348) -> (1/x=w349:dbl)
                n235 = Bundle By Name("Y"=w339, "dt"=w349) -> (w356:waveform(dbl))  [unwired: 1 in]
                n236 = Bundle By Name("Y"=w341, "dt"=w349) -> (w351:waveform(dbl))  [unwired: 1 in]
                n237 = Bundle By Name("Y"=w340, "dt"=w349) -> (w350:waveform(dbl))  [unwired: 1 in]
              }
              frame False {
                # "Sinusoid configurations"
                n238 = local read "reset\nphase?"() -> (w536:bool)
                n239 = local read "Frequency (Hz)"() -> (w537:dbl)
                n240 = local read "Amplitude (V)"() -> (w538:dbl)
                n241 = local read "Sine phase"() -> (w542:dbl)
                n242 = local write "Offset 2"("Offset") -> ()
                n243 = Subtract(x=w542, y=120.0) -> (x-y=w544:dbl)
                n244 = call <vilib>:"Sine Waveform.vi"("offset"="Offset", "sampling info"=w521, "reset signal"=w536, "phase"=w542, "amplitude"=w538, "frequency"=w537) -> ("signal out"=w526:waveform(dbl))  [unwired: 4 in, 1 out]
                n245 = Subtract(x=w542, y=240.0) -> (x-y=w541:dbl)
                n246 = call <vilib>:"Sine Waveform.vi"("offset"="Offset", "sampling info"=w521, "reset signal"=w536, "phase"=w544, "amplitude"=w538, "frequency"=w537) -> ("signal out"=w525:waveform(dbl))  [unwired: 4 in, 1 out]
                n247 = call <vilib>:"Sine Waveform.vi"("offset"="Offset", "sampling info"=w521, "reset signal"=w536, "phase"=w541, "amplitude"=w538, "frequency"=w537) -> ("signal out"=w524:waveform(dbl))  [unwired: 4 in, 1 out]
                n248 = case shown="\"R\"" "Fase ref" {
                  tunnel: w526 -> [_ _ w549]
                  tunnel: w525 -> [w547 _ _]
                  tunnel: w524 -> [_ w548 _]
                  tunnel: [w547 w548 w549] -> w523
                  frame "S" {
                  }
                  frame "T" {
                  }
                  frame "R" {
                  }
                }
                n249 = local read "Harmonics\nauto variation"() -> (w532:bool)
                n250 = local read "Amplitude (V)"() -> (w531:dbl)
                n251 = Or(x=w532, y="Harmonics") -> (x .or. y?=w534:bool)
                n252 = case shown="True" w534 {
                  tunnel: w524 -> [w572 w585]
                  tunnel: [w572 w584] -> w546
                  tunnel: w521 -> [_ w583]
                  tunnel: w525 -> [w571 w581]
                  tunnel: w526 -> [w570 w580]
                  tunnel: [w571 w578] -> w540
                  tunnel: [w570 w577] -> w539
                  tunnel: [w569 w574] -> w535
                  tunnel: w531 -> [w569 w574]
                  frame False {
                  }
                  frame True {
                    n253 = local read "Amplitude (%)"() -> (w576:dbl)
                    n254 = local read "Harmonic order"() -> (w582:i32)
                    n255 = local read "Frequency (Hz)"() -> (w575:dbl)
                    n256 = Divide(x=w576, y=100.0) -> (x/y=w587:dbl)
                    n257 = Multiply(x=w575, y=w582) -> (x*y=w590:dbl)
                    "Frequency" <- w590
                    n258 = Multiply(x=w574, y=w587) -> (x*y=w586:dbl)
                    n259 = call <vilib>:"Sine Waveform.vi"("sampling info"=w583, "phase"=180.0, "amplitude"=w586, "frequency"=w590) -> ("error out"=w573:errorcluster, "signal out"=w579:waveform(dbl))  [unwired: 6 in]
                    n260 = Add(1:w579, 2:w580, 4:w573) -> (0:w577:waveform(dbl))  [unwired: 1 out]
                    n261 = Add(1:w579, 2:w581, 4:w573) -> (0:w578:waveform(dbl))  [unwired: 1 out]
                    n262 = Add(1:w579, 2:w585, 4:w573) -> (0:w584:waveform(dbl))  [unwired: 1 out]
                  }
                }
                n263 = local read "Interference\nauto variation"() -> (w528:bool)
                n264 = Or(x="Interference", y=w528) -> (x .or. y?=w530:bool)
                n265 = case shown="True" w530 {
                  tunnel: w535 -> [_ w565]
                  tunnel: w521 -> [_ w564]
                  tunnel: w546 -> [w552 w563]
                  tunnel: [w552 w562] -> w520
                  tunnel: w540 -> [w551 w561]
                  tunnel: w539 -> [w550 w559]
                  tunnel: [w551 w560] -> w519
                  tunnel: [w550 w557] -> w518
                  frame False {
                  }
                  frame True {
                    n266 = local read "Interf.\nFrequency (Hz)"() -> (w555:dbl)
                    n267 = local read "Interf.\nAmplitude (%)"() -> (w556:dbl)
                    n268 = Divide(x=w556, y=100.0) -> (x/y=w567:dbl)
                    n269 = Multiply(x=w565, y=w567) -> (x*y=w566:dbl)
                    n270 = call <vilib>:"Sine Waveform.vi"("sampling info"=w564, "phase"=0.0, "amplitude"=w566, "frequency"=w555) -> ("error out"=w553:errorcluster, "signal out"=w558:waveform(dbl))  [unwired: 6 in]
                    n271 = Add(1:w558, 2:w561, 4:w553) -> (0:w560:waveform(dbl))  [unwired: 1 out]
                    n272 = Add(1:w558, 2:w559, 4:w553) -> (0:w557:waveform(dbl))  [unwired: 1 out]
                    n273 = Add(1:w558, 2:w563, 4:w553) -> (0:w562:waveform(dbl))  [unwired: 1 out]
                  }
                }
              }
            }
            n274 = case shown="True" "Noise" {
              tunnel: w283 -> [w316 w332]
              tunnel: w280 -> [w317 w331]
              tunnel: [w317 w330] -> w270
              tunnel: [w316 w329] -> w271
              tunnel: [w315 w328] -> w272
              tunnel: w282 -> [w315 w327]
              tunnel: w268 -> [_ w323]
              frame False {
              }
              frame True {
                # "Noise configurations"
                n275 = Square Root(x=2.0 ("offset")) -> (sqrt(x)=w320:dbl)
                n276 = Divide(x="Amplitude", y=w320) -> (x/y=w318:dbl)
                n277 = Bundle("Sampling rate"=w323, "Sampling rate"=w323) -> (w326:T11)  [unwired: 1 in]
                n278 = call <vilib>:"Tones and Noise Waveform.vi"("sampling info"=w326, "offset"=0.0, "noise (rms)"=w318, "tones"=T1 [{"frequency"=0.0, "amplitude"=0.0, "phase"=0.0}, {"frequency"=0.0, "amplitude"=0.0, "phase"=0.0}]) -> ("signal out"=w322:waveform(dbl))  [unwired: 6 in, 1 out]
                n279 = Add(1:w322, 2:w327) -> (0:w328:waveform(dbl))  [unwired: 1 in, 1 out]
                n280 = Add(1:w322, 2:w331) -> (0:w330:waveform(dbl))  [unwired: 1 in, 1 out]
                n281 = Add(1:w322, 2:w332) -> (0:w329:waveform(dbl))  [unwired: 1 in, 1 out]
              }
            }
            n282 = case shown="False" "Multi-freq. ?" {
              tunnel: w270 -> [w296 w310]
              tunnel: w272 -> [w295 w309]
              tunnel: [w295 w307] -> w273
              tunnel: [w294 w306] -> w274
              tunnel: [w296 w305] -> w275
              tunnel: w271 -> [w294 w304]
              tunnel: w268 -> [_ w302]
              tunnel: [w292 w301] -> w267
              tunnel: [w293 w298] -> w266
              tunnel: w265 -> [w292 _]
              frame False {
                n283 = local read "Frequency (Hz)"() -> (w293:dbl)
              }
              frame True {
                # "para gerar referencias"
                n284 = Square Root(x=2.0 ("offset")) -> (sqrt(x)=w314:dbl)
                n285 = Bundle("Sampling rate"=w302, "Sampling rate"=w302) -> (w303:T11)  [unwired: 1 in]
                n286 = Divide(x=0.0, y=w314) -> (x/y=w312:dbl)
                n287 = call <vilib>:"Tones and Noise Waveform.vi"("sampling info"=w303, "noise (rms)"=w312, "tones"="tones") -> ("error out"=w308:errorcluster, "signal out"=w301:waveform(dbl))  [unwired: 7 in]
                n288 = Index Array(array="tones", index=0) -> (element=w299:T12)
                n289 = Add(1:w301, 2:w310, 4:w308) -> (0:w305:waveform(dbl))  [unwired: 1 out]
                n290 = Add(1:w301, 2:w304, 4:w308) -> (0:w306:waveform(dbl))  [unwired: 1 out]
                n291 = Add(1:w301, 2:w309, 4:w308) -> (0:w307:waveform(dbl))  [unwired: 1 out]
                n292 = Unbundle By Name(w299) -> ("frequency"=w298:dbl)
              }
            }
          }
          frame #2 {
            # "Sinusoid > Channel 3"
            n293 = case shown="False" w596 {
              tunnel: [w631 w646] -> w606
              tunnel: [w630 w633] -> w612
              tunnel: w611 -> [_ w645]
              tunnel: [w629 w644] -> w594
              tunnel: w592 -> [_ w639]
              tunnel: w608 -> [w631 _]
              tunnel: w595 -> [w629 _]
              tunnel: w607 -> [w630 _]
              tunnel: w591 -> [_ w632]
              frame True {
              }
              frame False {
                w660 = 1000
                # "others phases"
                # "first phase"
                # "decimacao"
                n294 = Unbundle By Name(w639) -> ("Y"=w640:dbl[], "dt"=w641:dbl)
                n295 = Divide(x=w645, y=w660) -> (x/y=w659:dbl)
                n296 = Multiply(x=w659, y=w641) -> (x*y=w662:dbl)
                n297 = for {
                  N: w660 -> [_]
                  tunnel: w640 -> [w678]
                  tunnel: [w675] -> w663 mode=indexing
                  tunnel: w659 -> [w674]
                  i -> [w676]
                  n298 = Multiply(x=w676, y=w674) -> (x*y=w677:dbl)
                  n299 = Index Array(array=w678, index=w677) -> (element=w675:dbl)
                }
                n300 = local read "Pulse frequency"() -> (w650:dbl)
                n301 = Subtract(x=w632, y=50.0) -> (x-y=w653:dbl)
                n302 = Bundle By Name("Y"=w663, "dt"=w662) -> (w661:waveform(dbl))  [unwired: 1 in]
                n303 = Multiply(x=w653, y=360.0) -> (x*y=w652:dbl)
                n304 = call-poly <vilib>:"Extract Single Tone Information.vi"("time signal in"=w661) -> ("detected phase (deg)"=w657:dbl)  [unwired: 5 in, 5 out]
                n305 = Divide(x=w652, y=w650) -> (x/y=w649:dbl)
                n306 = Subtract(x=w657, y=90.0) -> (x-y=w656:dbl)
                n307 = local read "Amplitude (V)"() -> (w643:dbl)
                n308 = local read "Frequency (Hz)"() -> (w642:dbl)
                n309 = call "angle_corrector.vi"("angle"=w656) -> ("angle corrected"=w647:dbl)  [unwired: 10 in]
                "Phase (deg)" <- w647
                n310 = for {
                  N: w650 -> [_]
                  tunnel: [w667] -> w651 mode=indexing
                  tunnel: w649 -> [w671]
                  tunnel: w647 -> [w672]
                  tunnel: w643 -> [w669]
                  tunnel: [w669] -> w646 mode=indexing
                  tunnel: w642 -> [w668]
                  tunnel: [w668] -> w644 mode=indexing
                  i -> [w673]
                  n311 = Multiply(x=w671, y=w673) -> (x*y=w670:dbl)
                  n312 = Add(x=w672, y=w670) -> (x+y=w666:dbl)
                  n313 = call "angle_corrector2.vi"("angle"=w666) -> ("angle corrected"=w667:dbl)  [unwired: 10 in]
                }
                n314 = local read "phase 2"() -> (w636:dbl)
                n315 = Replace Array Subset(array=w651, new element=w647, index=0) -> (w637:dbl[])
                n316 = Multiply(x=w636, y=-2.0) -> (x*y=w635:dbl)
                n317 = Add(x=w637, y=w635) -> (x+y=w634:dbl[])
                n318 = for {
                  tunnel: w634 -> [w665] mode=indexing
                  tunnel: [w664] -> w633 mode=indexing
                  n319 = call "angle_corrector_array.vi"("angle"=w665) -> ("angle corrected"=w664:dbl)  [unwired: 10 in]
                }
              }
            }
            n320 = Unbundle By Name(w605) -> ("Y"=w601:dbl[])
            n321 = Unbundle By Name(w604) -> ("Y"=w602:dbl[])
            n322 = Unbundle By Name(w599) -> ("Y"=w597:dbl[])
            n323 = Unbundle By Name(w598) -> ("Y"=w600:dbl[])
            n324 = case shown="True" "Boolean" {
              tunnel: w611 -> [_ w624]
              tunnel: w610 -> [_ w623]
              tunnel: w597 -> [_ w622]
              tunnel: w600 -> [_ w621]
              frame False {
              }
              frame True {
                w620 = 0 ("start index (0)")
                # "First cycle visualization"
                n325 = Divide(x=w624, y=w623) -> (x/y=w627:dbl)
                n326 = To Long Integer(number=w627) -> (32bit integer=w625:i32)
                n327 = Search 1D Array(1D array=w621, element=2.95, start index (0)=w620) -> ()  [unwired: 1 out]
                n328 = Array Subset(array=w622, index=w620, length=w625) -> (→"Cycle visualization":dbl[])
              }
            }
            n329 = Build Array(w600, w597, w601, w602) -> (w609:dbl[][])
            n330 = for {
              tunnel: w594 -> [w616] mode=indexing
              shift-right: [w616] -> _
              shift-left: _ -> [w619]
              tunnel: [w615] -> w593 mode=indexing
              n331 = local read "Pulse frequency"() -> (w617:dbl)
              n332 = Subtract(x=w616, y=w619) -> (x-y=w618:dbl)
              n333 = Multiply(x=w618, y=w617) -> (x*y=w615:dbl)
            }
          }
          frame #3 {
            n334 = case shown="0, Default" w680 {
              tunnel: w679 -> [w685 w686]
              frame 0, Default {
                "rocof0" <- w685
              }
              frame 1 {
                "rocof1" <- w686
              }
            }
            n335 = case shown="1" w680 {
              tunnel: w681 -> [w687 w688]
              frame 0, Default {
                "freq0" <- w687
              }
              frame 1 {
                "freq1" <- w688
              }
            }
            n336 = case shown="1" w680 {
              tunnel: w682 -> [w689 w690]
              frame 0, Default {
                "magnitude0" <- w689
              }
              frame 1 {
                "magnitude1" <- w690
              }
            }
            n337 = case shown="0, Default" w680 {
              tunnel: w683 -> [w691 w692]
              frame 0, Default {
                "phases0" <- w691
              }
              frame 1 {
                "phases1" <- w692
              }
            }
          }
        }
        n338 = call-poly <vilib>:"DAQmx Write.vi"("task/channels in"=w76, "data"=w74, "error in"=w93) -> ("task out"=w91:refnum<k21>, "error out"=w92:errorcluster)  [unwired: 10 in, 1 out]
        n339 = node-c288() -> ()  [unwired: 5 in, 1 out]
      }
      n340 = call <vilib>:"DAQmx Stop Task.vi"("task/channels in"=w53, "error in"=w54) -> ("task out"=w60:refnum<k21>, "error out"=w39:errorcluster)  [unwired: 12 in]
      n341 = node-c288(w68) -> (→"Iteration Duration":i64)  [unwired: 6 out]
      n342 = call <vilib>:"DAQmx Clear Task.vi"("task in"=w60, "error in"=w39) -> ("error out"=w63:errorcluster)  [unwired: 13 in]
      n343 = call <vilib>:"Simple Error Handler.vi"("type of dialog (OK msg:1)"=w65, "error in (no error)"=w63) -> ()  [unwired: 3 in, 5 out]
    }
  }
  n344 = Build Array("Loop1", "Loop2") -> (w4:string[])
  n345 = call <vilib>:"Synchronize Timed Structure Starts.vi"("timed structure names"=w4, "synchronization group name"="grupo de sincronismo") -> ()  [unwired: 8 in, 2 out]
  n346 = case shown="True" "Serial communication" {
    selector: "Serial communication" -> [_ w709]
    tunnel: "Loop2" -> [_ w710]
    frame False {
    }
    frame True {
      n347 = case shown="True" w709 {
        tunnel: [_ w744] -> w727
        tunnel: [_ w736] -> w726
        frame False {
        }
        frame True {
          n348 = call-poly "VISA Configure Serial Port"("VISA resource name"="Porta", "timeout (10sec)"="timeout (ms)", "Enable Termination\nChar (T)"=FALSE ("Enable Termination\nChar (T)"), "baud rate (9600)"="baud rate (kB)", "data bits (8)"="data bits (8)", "parity (0:none)"="parity (0:none)", "stop bits (10: 1 bit)"="stop bits (10: 1 bit)", "flow control (0:none)"="flow control (0:none)") -> ("VISA resource name out"=w744:refnum<visa-resource-name>, "error out"=w736:errorcluster)  [unwired: 6 in]
        }
      }
      n349 = call-poly <vilib>:"DAQmx Create Timing Source.vi"("counter"=tag "Dev1/ctr0", "frequency"=1000.0) -> ("timing source out"=w712:string)  [unwired: 12 in, 1 out]
      n350 = Build Path(base path="Directory", name or relative path="File name") -> (appended path=w714:path)
      n351 = node-c288(w712, i64 0 ("Period"), 100 ("Priority"), 1 ("Processor"), w710, nitl_modes."Process missed periods, ignore original phase" ("Mode"), i64 40 ("Offset")) -> (w734:T8)  [unwired: 2 in]
      n352 = Open/Create/Replace File(file path (use dialog)=w714, operation (0:open)=T13."replace or create", access (0:read/write)=enum16{"read/write", "read-only", "write-only"}."write-only") -> (refnum out=w717:refnum<file>, error out=w718:errorcluster)  [unwired: 3 in, 1 out]
      n353 = timed-loop {
        timing: w734 -> [_]
        timing-out: [_] -> w733
        tunnel: w726 -> [w817]
        tunnel: w727 -> [w816]
        tunnel: [w815] -> w725
        tunnel: [w814] -> w724
        shift-right: [w813] -> _
        shift-left: 0 ("t") -> [w812]
        shift-right: [w776] -> _
        shift-left: 0 ("initial phase") -> [w777]
        tunnel: [w766] -> w722
        tunnel: [w765] -> w721
        tunnel: w718 -> [w764]
        tunnel: w717 -> [w763]
        tunnel: "frames per second" -> [w745]
        i -> [w774]
        stop <- "stop" stop-if-true
        n354 = node-c288() -> (w798:errorcluster, →"Iteration Duration 2":i64)  [unwired: 1 in, 2 out]
        n355 = flat-sequence {
          tunnel: w816 -> [w882]
          tunnel: w817 -> [w883]
          tunnel: [w883] -> w794
          tunnel: [w882] -> w792
          tunnel: w812 -> [w878]
          tunnel: [w873] -> w793
          tunnel: w745 -> [w869]
          tunnel: [w904] -> w791
          tunnel: [w902] -> w790
          tunnel: [w895] -> w789
          tunnel: [w893] -> w795
          tunnel: [w910] -> w788
          tunnel: [w894] -> w796
          tunnel: [w911] -> w787
          tunnel: [w909] -> w797
          tunnel: w777 -> [w898]
          tunnel: w793 -> [w900]
          tunnel: w792 -> [w907]
          tunnel: w794 -> [w908]
          tunnel: [w891] -> w758
          tunnel: [w897] -> w753
          tunnel: w791 -> [w946]
          tunnel: w790 -> [w945]
          tunnel: w789 -> [w931]
          tunnel: w795 -> [w932]
          tunnel: w788 -> [w933]
          tunnel: w796 -> [w936]
          tunnel: w787 -> [w929]
          tunnel: w797 -> [w927]
          tunnel: [w946] -> w815
          tunnel: [w945] -> w814
          tunnel: [w935] -> w768
          tunnel: [w928] -> w769
          tunnel: [w934] -> w770
          tunnel: [w933] -> w771
          tunnel: [w930] -> w772
          tunnel: [w927] -> w773
          tunnel: [w925] -> w752
          tunnel: w758 -> [w926]
          tunnel: w753 -> [w924]
          tunnel: [w924] -> w751
          frame #0 {
            n356 = To Long Integer(number=w869) -> (32bit integer=w870:i32)
            n357 = Multiply(x=2 ("y"), y=w870) -> (x*y=w871:i32)
            n358 = Greater Or Equal?(x=w878, y=w870) -> (x >= y?=w877:bool)
            n359 = Greater Or Equal?(x=w878, y=w871) -> (x >= y?=w876:bool)
            n360 = Select(t=1, s=w877, f=0) -> (s? t:f=w874:i32)
            n361 = Wait (ms)(milliseconds to wait=u32 1) -> ()  [unwired: 1 out]
            n362 = Select(t=2, s=w876, f=w874) -> (s? t:f=w873:i32)
          }
          frame #1 {
            (unwired) "0" ("read buffer")
            # "leituras"
            # "Conversor"
            n363 = VISA Flush I/O Buffer(VISA resource name=w907, error in (no error)=w908) -> (VISA resource name out=w901:refnum<visa-resource-name>, error out=w905:errorcluster)  [unwired: 1 in]
            n364 = case shown="1" w900 {
              tunnel: [w919 w920] -> w913
              frame 0, Default {
                n365 = local read "magnitude0"() -> (w919:dbl[])
              }
              frame 1 {
                n366 = local read "magnitude1"() -> (w920:dbl[])
              }
            }
            n367 = case shown="1" w900 {
              tunnel: [w921 w922] -> w914
              frame 0, Default {
                n368 = local read "phases0"() -> (w921:dbl[])
              }
              frame 1 {
                n369 = local read "phases1"() -> (w922:dbl[])
              }
            }
            n370 = case shown="0, Default" w900 {
              tunnel: [w915 w916] -> w899
              frame 0, Default {
                n371 = local read "rocof0"() -> (w915:dbl[])
              }
              frame 1 {
                n372 = local read "rocof1"() -> (w916:dbl[])
              }
            }
            n373 = case shown="0, Default" w900 {
              tunnel: [w917 w918] -> w912
              frame 0, Default {
                n374 = local read "freq0"() -> (w917:dbl[])
              }
              frame 1 {
                n375 = local read "freq1"() -> (w918:dbl[])
              }
            }
            n376 = VISA Read(VISA resource name=w901, byte count="byte count", error in (no error)=w905) -> (VISA resource name out=w902:refnum<visa-resource-name>, read buffer=w903:string, error out=w904:errorcluster)  [unwired: 1 out]
            n377 = String To Byte Array(string=w903) -> (unsigned byte array=w896:u8[])
            n378 = Index Array(array=w913, index=w898) -> (element=w911:dbl)
            n379 = Index Array(array=w899, index=w898) -> (element=w897:dbl)
            n380 = Index Array(array=w912, index=w898) -> (element=w909:dbl)
            n381 = Index Array(array=w914, index=w898) -> (element=w910:dbl)
            n382 = call "Conversor_float.vi"("subarray"=w896) -> ("Dados"=w892:sgl[])  [unwired: 5 in]
            "data" <- w892
            n383 = Multiply(x="Index component", y=1) -> (x*y=w886:i32)
            n384 = Increment(x=w886) -> (x+1=w890:i32)
            n385 = Increment(x=w890) -> (x+1=w889:i32)
            n386 = Increment(x=w889) -> (x+1=w888:i32)
            n387 = Index Array(array=w892, index=w890) -> (element=w894:sgl)
            n388 = Index Array(array=w892, index=w886) -> (element=w895:sgl)
            n389 = Index Array(array=w892, index=w889) -> (element=w893:sgl)
            n390 = Index Array(array=w892, index=w888) -> (element=w891:sgl)
            "read buffer" <- ""
          }
          frame #2 {
            # "correçoes"
            n391 = To Double Precision Float(number=w932) -> (double precision float=w937:dbl)
            n392 = To Double Precision Float(number=w926) -> (double precision float=w925:dbl)
            n393 = case shown="False" "RMS?" {
              tunnel: w929 -> [w947 w949]
              tunnel: [w947 w948] -> w928
              frame False {
              }
              frame True {
                n394 = Square Root(x=2.0) -> (sqrt(x)=w951:dbl)
                n395 = Divide(x=w949, y=w951) -> (x/y=w948:dbl)
              }
            }
            n396 = Add(x=w937, y="Frequency\noff-set") -> (x+y=w930:dbl)
            n397 = To Double Precision Float(number=w931) -> (double precision float=w939:dbl)
            n398 = To Double Precision Float(number=w936) -> (double precision float=w938:dbl)
            n399 = Add(x=w938, y="Angle\noff-set") -> (x+y=w934:dbl)
            n400 = Multiply(x=w939, y="Magnitude\ncoefficient") -> (x*y=w941:dbl)
            n401 = Add(x=w941, y="Magnitude\noff-set") -> (x+y=w935:dbl)
          }
        }
        n402 = Multiply(x=w745, y=u16 2) -> (x*y=w806:dbl)
        n403 = Decrement(x=w806) -> (x-1=w805:dbl)
        n404 = Equal?(x=w805, y=w812) -> (x = y?=w803:bool)
        n405 = Increment(x=w812) -> (x+1=w802:i32)
        n406 = Select(t=0, s=w803, f=w802) -> (s? t:f=w813:i32)
        n407 = local read "Pulse frequency"() -> (w800:dbl)
        n408 = Decrement(x=w800) -> (x-1=w801:dbl)
        n409 = Equal?(x=w777, y=w801) -> (x = y?=w808:bool)
        n410 = Increment(x=w777) -> (x+1=w810:i32)
        n411 = Select(t=u16 0, s=w808, f=w810) -> (s? t:f=w776:i32)
        n412 = case shown="True" "Data save" {
          tunnel: w768 -> [_ w838]
          tunnel: w770 -> [_ w837]
          tunnel: w772 -> [_ w835]
          tunnel: w773 -> [_ w834]
          tunnel: w774 -> [_ w830]
          tunnel: w771 -> [_ w836]
          tunnel: w769 -> [_ w831]
          tunnel: [_ w829] -> w767
          tunnel: w752 -> [_ w828]
          tunnel: w751 -> [_ w827]
          frame False {
          }
          frame True {
            n413 = local read "Multi-freq. ?"() -> (w825:bool)
            n414 = feedback #12(w830) -> (w833:i32)
            n415 = feedback-in #12(w833) -> ()
            n416 = Not(x=w825) -> (.not. x?=w826:bool)
            n417 = Subtract(x=w830, y=w833) -> (x-y=w832:i32)
            n418 = case shown="True" w826 {
              tunnel: w838 -> [_ w862]
              tunnel: w837 -> [_ w861]
              tunnel: w836 -> [_ w860]
              tunnel: w835 -> [_ w859]
              tunnel: w834 -> [_ w858]
              tunnel: w832 -> [w840 w857]
              tunnel: w831 -> [_ w856]
              tunnel: [w843 w854] -> w829
              tunnel: w828 -> [_ w853]
              tunnel: w827 -> [_ w852]
              frame False {
                n419 = local read "data"() -> (w845:sgl[])
                n420 = for {
                  tunnel: w845 -> [w850] mode=indexing
                  shift-right: [w847] -> w841
                  shift-left: "" -> [w846]
                  n421 = Number To Fractional String(number=w850) -> (F-format string=w849:string)  [unwired: 3 in]
                  n422 = Concatenate Strings(w849, "\t", w846) -> (w847:string)
                }
                n423 = Format Into String(w840, "\t", w841, "\r\n") -> (resulting string=w843:string)  [unwired: 3 in, 1 out]
              }
              frame True {
                w855 = "\t"
                n424 = Format Into String(w857, w855, w862, w855, w856, w855, w861, w855, w860, w855, w859, w855, w858, w855, w853, w855, w852, "\r\n") -> (resulting string=w854:string)  [unwired: 3 in, 1 out]
              }
            }
          }
        }
        n425 = Initialize Array(w768, 1 ("dimension size")) -> (w755:dbl[])
        "Voltage measured" <- w755
        n426 = Initialize Array(w769, 1 ("dimension size")) -> (w756:dbl[])
        "Voltage reference" <- w756
        n427 = Initialize Array(w770, 1 ("dimension size")) -> (w746:dbl[])
        "Angle measured" <- w746
        n428 = Initialize Array(w771, 1 ("dimension size")) -> (w747:dbl[])
        "Angle reference" <- w747
        n429 = case shown="True" "?" {
          tunnel: w755 -> [_ w961]
          tunnel: w756 -> [_ w960]
          frame False {
          }
          frame True {
            n430 = Build Array(w961, w960) -> (w963:dbl[][])
            n431 = Transpose 2D Array(2D array=w963) -> (transposed array=→"Magnitude measures (V)":dbl[][])
          }
        }
        n432 = case shown="True" "?" {
          tunnel: w747 -> [_ w956]
          tunnel: w746 -> [_ w957]
          frame False {
          }
          frame True {
            n433 = Build Array(w957, w956) -> (w959:dbl[][])
            n434 = Transpose 2D Array(2D array=w959) -> (transposed array=→"Phase measures (º)":dbl[][])
          }
        }
        n435 = Write to Text File(file (use dialog)=w763, text=w767, error in=w764) -> (refnum out=w765:refnum<file>, error out=w766:errorcluster)  [unwired: 1 in, 1 out]
        n436 = Initialize Array(w772, 1 ("dimension size")) -> (w748:dbl[])
        "Frequency measured" <- w748
        n437 = Initialize Array(w773, 1 ("dimension size")) -> (w749:dbl[])
        "Frequency reference" <- w749
        n438 = Initialize Array(w752, 1 ("dimension size")) -> (w754:dbl[])
        "ROCOF measured" <- w754
        n439 = Initialize Array(w751, 1 ("dimension size")) -> (w759:dbl[])
        "ROCOF reference" <- w759
        n440 = case shown="True" "Boolean 3" {
          tunnel: w756 -> [_ w864]
          tunnel: w755 -> [_ w866]
          tunnel: w746 -> [_ w865]
          tunnel: w747 -> [_ w863]
          frame False {
          }
          frame True {
            n441 = call-poly <vilib>:"Plot Helper.vi"("radius vector"=w866, "theta vector"=w865) -> ("2D Plot Class Obj Array out"=w867:refnum<class "2D Plot Datatype.lvclass">[])  [unwired: 2 in, 7 out]
            n442 = call-poly <vilib>:"Plot Helper.vi"("radius vector"=w864, "theta vector"=w863, "2D Plot Class Obj Array in"=w867) -> ("2D Plot Class Obj Array out"=→"Phasors visualization":refnum<class "2D Plot Datatype.lvclass">[])  [unwired: 1 in, 7 out]
          }
        }
        n443 = case shown="True" "?" {
          tunnel: w754 -> [_ w822]
          tunnel: w759 -> [_ w821]
          frame False {
          }
          frame True {
            n444 = Build Array(w822, w821) -> (w823:dbl[][])
            n445 = Transpose 2D Array(2D array=w823) -> (transposed array=→"ROCOF (Hz/s)":dbl[][])
          }
        }
        n446 = case shown="True" "?" {
          tunnel: w747 -> [_ w820]
          tunnel: w746 -> [_ w819]
          frame False {
          }
          frame True {
            n447 = Subtract(x=w820, y=w819) -> (x-y=→"Phase measures (º) 2":dbl[])
          }
        }
        n448 = case shown="True" "?" {
          tunnel: w749 -> [_ w954]
          tunnel: w748 -> [_ w953]
          frame False {
          }
          frame True {
            n449 = Build Array(w953, w954) -> (w955:dbl[][])
            n450 = Transpose 2D Array(2D array=w955) -> (transposed array=→"Frequency measures (Hz)":dbl[][])
          }
        }
        n451 = node-c288(w798) -> ()  [unwired: 1 out]
      }
      n452 = node-c288(w733) -> ()  [unwired: 1 out]
      n453 = Close File(refnum=w721, error in=w722) -> ()  [unwired: 2 out]
      n454 = VISA Close(VISA resource name=w724, error in (no error)=w725) -> ()  [unwired: 1 out]
    }
  }
  n455 = case shown="True" TRUE {
    frame False {
    }
    frame True {
      n456 = while {
        stop <- FALSE stop-if-true
        n457 = case shown="\"Real-Time Data\"" "Tab Control" {
          frame "Communication", Default {
          }
          frame "Real-Time Data" {
            n458 = local read "Pulse frequency"() -> (w984:dbl)
            n459 = Initialize Array(0.0 ("element"), w984) -> (w983:dbl[])
            "initialized array" <- w983
            n460 = while {
              shift-right: [w1023] -> _
              shift-left: 0 -> [w1000]
              tunnel: w984 -> [w1022]
              tunnel: w983 -> [w997]
              stop <- w1013 stop-if-true
              # "Escrevem nos controles da  aba principal"
              # "Controles da aba Real-Time Data"
              # "Indicadores da aba Real-Time Data"
              n461 = local read "Phase (deg)"() -> (→"Phase (degrees) 2":dbl)
              n462 = Wait (ms)(milliseconds to wait=u32 30) -> ()  [unwired: 1 out]
              n463 = local read "ROCOF measured"() -> (w998:dbl[])
              n464 = local read "ROCOF reference"() -> (w999:dbl[])
              n465 = local read "Frequency reference"() -> (w1006:dbl[])
              n466 = local read "Voltage measured"() -> (w994:dbl[])
              n467 = local read "Frequency measured"() -> (w1005:dbl[])
              n468 = local read "Angle measured"() -> (w1003:dbl[])
              n469 = local read "Angle reference"() -> (w1004:dbl[])
              n470 = local read "Voltage reference"() -> (w993:dbl[])
              n471 = Equal?(x=w1022, y=w1000) -> (x = y?=w1014:bool)
              n472 = Increment(x=w1000) -> (x+1=w1025:i32)
              n473 = feedback #13(w997) -> (w1031:dbl[])
              n474 = Replace Array Subset(array=w1031, new element=w993, index=w1000) -> (w1017:dbl[])
              n475 = feedback-in #13(w1017) -> ()
              n476 = feedback #14(w997) -> (w1030:dbl[])
              n477 = Replace Array Subset(array=w1030, new element=w994, index=w1000) -> (w1018:dbl[])
              n478 = feedback-in #14(w1018) -> ()
              n479 = feedback #15(w997) -> (w1027:dbl[])
              n480 = Replace Array Subset(array=w1027, new element=w1005, index=w1000) -> (w1015:dbl[])
              n481 = feedback-in #15(w1015) -> ()
              n482 = feedback #16(w997) -> (w1026:dbl[])
              n483 = Replace Array Subset(array=w1026, new element=w1006, index=w1000) -> (w1016:dbl[])
              n484 = feedback-in #16(w1016) -> ()
              n485 = feedback #17(w997) -> (w1029:dbl[])
              n486 = Replace Array Subset(array=w1029, new element=w1003, index=w1000) -> (w1019:dbl[])
              n487 = feedback-in #17(w1019) -> ()
              n488 = feedback #18(w997) -> (w1028:dbl[])
              n489 = Replace Array Subset(array=w1028, new element=w1004, index=w1000) -> (w1020:dbl[])
              n490 = feedback-in #18(w1020) -> ()
              n491 = feedback #19(w997) -> (w1002:dbl[])
              n492 = Replace Array Subset(array=w1002, new element=w998, index=w1000) -> (w996:dbl[])
              n493 = feedback-in #19(w996) -> ()
              n494 = feedback #20(w997) -> (w1001:dbl[])
              n495 = Replace Array Subset(array=w1001, new element=w999, index=w1000) -> (w995:dbl[])
              n496 = feedback-in #20(w995) -> ()
              n497 = Select(t=0, s=w1014, f=w1025) -> (s? t:f=w1023:i32)
              n498 = case shown="True" w1014 {
                selector: w1014 -> [_ w1043]
                tunnel: w1020 -> [_ w1059]
                tunnel: w1019 -> [_ w1058]
                tunnel: w1018 -> [_ w1033]
                tunnel: w1017 -> [_ w1042]
                tunnel: w1016 -> [_ w1053]
                tunnel: w1015 -> [_ w1052]
                tunnel: [FALSE w1043] -> w1013
                tunnel: w996 -> [_ w1038]
                tunnel: w995 -> [_ w1037]
                frame False {
                }
                frame True {
                  n499 = call "Statistical measure - basics - 4.vi"("Data measured"=w1038, "Data reference"=w1037) -> ("Statistcs"=w1036:T14)  [unwired: 12 in, 1 out]
                  n500 = Add Array Elements(numeric array=w1033) -> (sum=w1041:dbl)
                  n501 = Array Size(array=w1033) -> (size(s)=w1040:i32)
                  n502 = call "Statistical measure - basics percentual - 1.vi"("Data measured"=w1042, "Data reference"=w1033) -> ("Statistcs"=w1054:T14)  [unwired: 12 in, 1 out]
                  n503 = call "Statistical measure - basics - 1.vi"("Data measured"=w1058, "Data reference"=w1059) -> ("Statistcs"=w1061:T14)  [unwired: 12 in, 1 out]
                  n504 = call "Statistical measure - basics - 3.vi"("Data measured"=w1052, "Data reference"=w1053) -> ("Statistcs"=w1051:T14)  [unwired: 12 in, 1 out]
                  n505 = call "TVE.vi"("Angle reference"=w1059, "Angle measured"=w1058, "Voltage reference"=w1033, "Voltage measured"=w1042) -> ("Array"=w1056:dbl[])
                  n506 = local read "initialized array"() -> (w1057:dbl[])
                  n507 = Unbundle By Name(w1036) -> ("max dev"=→"max rocof":dbl, "mean dev"=→"mean rocof":dbl)
                  n508 = Unbundle By Name(w1054) -> ("max dev"=→"max magnitude":dbl, "mean dev"=→"mean dev":dbl)
                  n509 = Divide(x=w1041, y=w1040) -> (x/y=→"Media":dbl)
                  n510 = Unbundle By Name(w1061) -> ("max dev"=→"max phase":dbl, "mean dev"=→"mean phase":dbl)
                  n511 = Unbundle By Name(w1051) -> ("max dev"=→"max freq":dbl, "mean dev"=→"mean freq":dbl)
                  n512 = call "Statistical measure - basics - 2.vi"("Data measured"=w1056, "Data reference"=w1057) -> ("Statistcs"=w1055:T14)  [unwired: 12 in, 1 out]
                  n513 = Unbundle By Name(w1055) -> ("max dev"=→"max tve":dbl, "mean dev"=→"mean tve":dbl)
                }
              }
              n514 = local write "Amplitude (%)"("Amp. (%) 2") -> ()
              n515 = local write "Interf.\nFrequency (Hz)"("Interf. Frequency 2") -> ()
              n516 = local write "Interf.\nAmplitude (%)"("amplitude") -> ()
              n517 = local write "Interference"("Interference 2") -> ()
              n518 = local write "Order"("Order 2") -> ()
              n519 = local write "Harmonics"("Harmonics 2") -> ()
              n520 = local write "Offset"("Offset 2") -> ()
              n521 = local write "Phase"("Phase 2") -> ()
              n522 = local write "Amplitude"("Amplitude 2") -> ()
              n523 = local write "Frequency"("Frequency 2") -> ()
              n524 = local write "reset\nphase?"("reset signal 2") -> ()
            }
          }
          frame "Measure statistics" {
          }
        }
        n525 = Wait (ms)(milliseconds to wait=u32 1000) -> ()  [unwired: 1 out]
      }
    }
  }
